vi "CDMA_TxSCH.vi"(7 "sc_group_num_tx":dbl, 8 "error in (no error)":errorcluster caption="错误输入（无错误）", 9 "Gs":dbl, 10 "Gp":dbl, 11 "Path":path) -> (0 "error out":errorcluster caption="错误输出", 3 "sch_data":cdb[](array[numeric]))   [LabVIEW 2015]
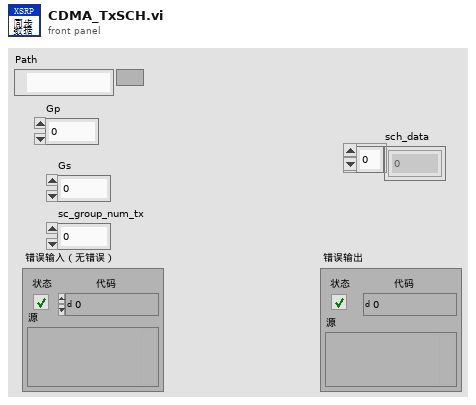
[diagram p1: front panel]
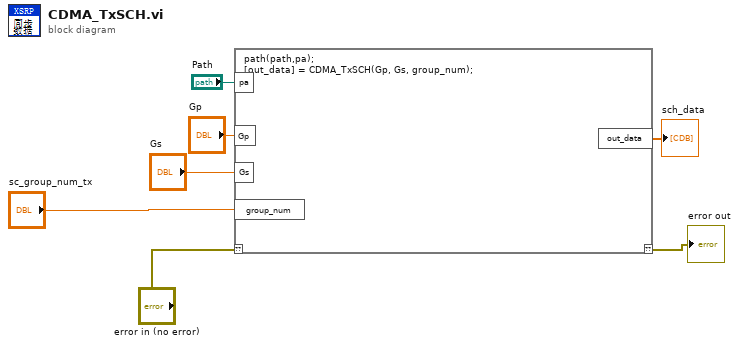
[diagram p0: block diagram]
diagram:
  n1 = script code="path(path,pa);\n[out_data] = CDMA_TxSCH(Gp, Gs, group_num);"("??"="error in (no error)", "pa"="Path", "Gp"="Gp", "Gs"="Gs", "group_num"="sc_group_num_tx") -> ("??"=→"error out":errorcluster, "out_data"=→"sch_data":cdb[])
